vi "Get Pane Ref.vi"(7 "VI Ref":refnum<vi>, 8 "Error":errorcluster, 11 "FP":refnum<class "FP.lvclass">) -> (0 "Error Out":errorcluster, 2 "Pane Ref Out":refnum<vi>, 3 "FP Out":refnum<class "FP.lvclass">, 5 "VI Ref Out":refnum<vi>)   [LabVIEW 2023, in "FP.lvclass"]
uses:
  FP.lvclass
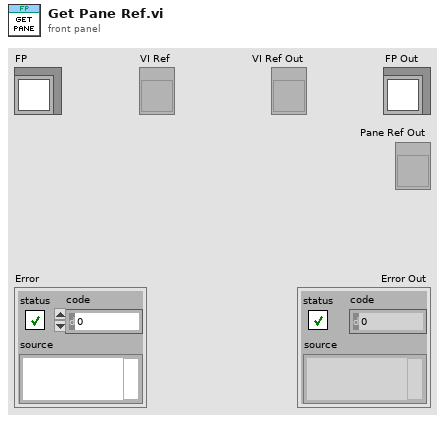
[diagram p1: front panel]
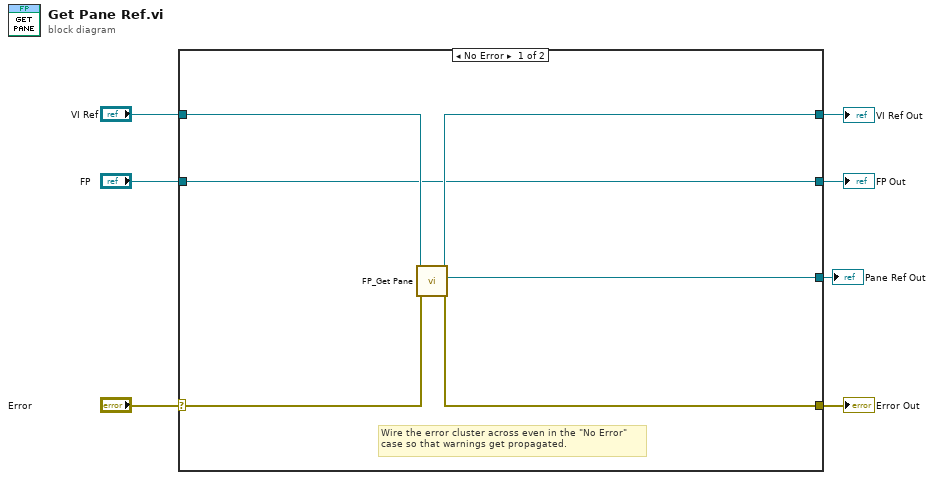
[diagram p0: block diagram]
diagram:
  n1 = case shown="No Error" "Error" {
    selector: "Error" -> [w9 w16]
    tunnel: [w8 w16] -> w6
    tunnel: [w11 w15] -> w4
    tunnel: "FP" -> [w11 w15]
    tunnel: "VI Ref" -> [w13 w14]
    tunnel: [w12 w14] -> w2
    tunnel: [w10 _] -> w1
    frame No Error {
      # "Wire the error cluster across even in the \"No Error\"\ncase so that warnings get propagated."
      n2 = call "FP_Get Pane.vi"("Error"=w9, "VI"=w13) -> ("Error Out"=w8:errorcluster, "Pane Refnum Out"=w10:refnum<vi>, "VI Out"=w12:refnum<vi>)  [unwired: 7 in]
    }
    frame Error {
    }
  }
  "Error Out" <- w6
  "FP Out" <- w4
  "VI Ref Out" <- w2
  "Pane Ref Out" <- w1
